vi "UI Main.vi"() -> ()   [LabVIEW 2012]
uses:
  controls/Control Configuration.ctl
  controls/UI Data.ctl
  controls/All FPGA Configuration Values.ctl
  controls/FPGA State.ctl
  controls/Raw Values.ctl
  Globals/Global - All UI Loop Stop.vi
  Globals/Global - UI Stream and Variable Connections.vi
  Globals/Global - Configuration Options.vi
  support/User Event - Stop/User Event - Stop.lvlib
  support/Message Queue/Message Queue.lvlib
panel:
  in  "Switch to Safe State":bool
  in  "Exit":bool
  out "System Status":string
  out "Current FPGA Control Mode":u16(ring) items=["Safe State", "Manual", "Control (PID)"]
  in  "Settings Tab":T1(tab)
  in  "Channel 3 Setpoint":fxp<+/-,16,5>
  in  "Channel 2 Setpoint":fxp<+/-,16,5>
  in  "Channel 1 Setpoint":fxp<+/-,16,5>
  in  "Channel 0 Setpoint":fxp<+/-,16,5>
  in  "Update Control Configuration":bool
  in  "Control Configurations":T2[](array[typedef])
  in  "Run Control":bool
  in  "Stop Control":bool
  in  "Channel 3 Manual Value":fxp<+/-,16,5>
  in  "Channel 2 Manual Value":fxp<+/-,16,5>
  in  "Channel 1 Manual Value":fxp<+/-,16,5>
  in  "Channel 0 Manual Value":fxp<+/-,16,5>
  in  "Run Manual":bool
  in  "Stop Manual":bool
  out "Input Values":T3(graph)
  out "Output Values":T3(graph)
  out "Actual Loop Period (ticks)":u32
  out "Largest Contiguous Memory (bytes)":dbl(graph)
  out "CPU Usage (%)":dbl(graph)
  out "Connected?":bool
  in  "Connect to Controller":bool
  in  "Controller Address":string
  # "LabVIEW FPGA Control on CompactRIO"
  # "Connection Settings"
  # "Element 0 - Chan 0\nElement 1 - Chan 1\nElement 2 - Chan 2\nElement 3 - Chan 3"
  # "Setpoint changes are sent to the target automatically."
  # "Control Configuration changes are sent to the target when you click \"Update Control Configurations\"."
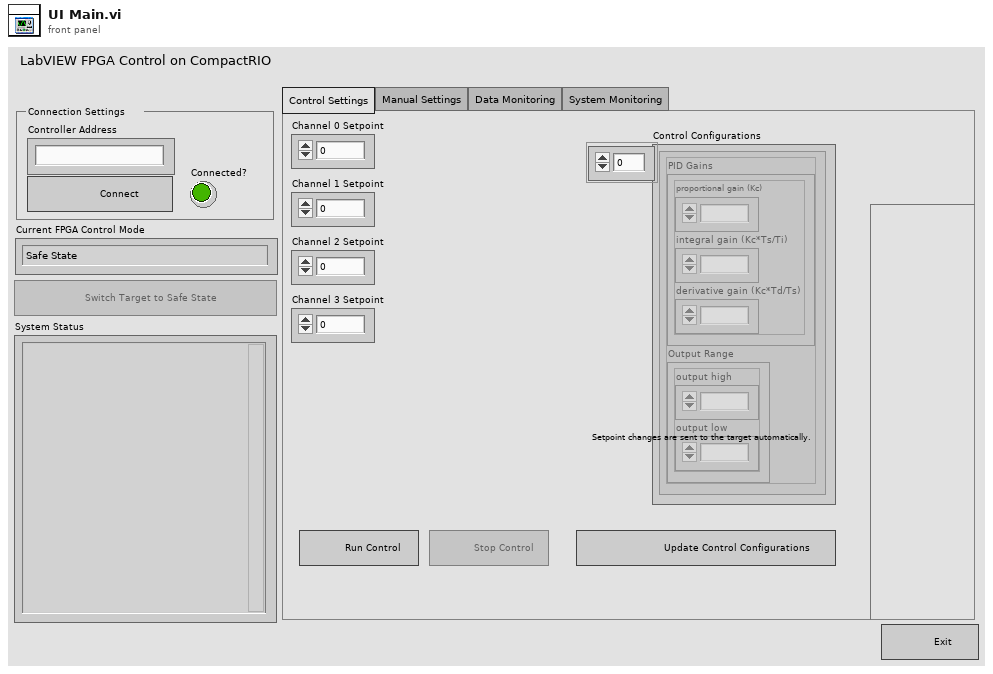
[diagram p1: front panel]
types:
  T1 = enum32{"Control Settings", "Manual Settings", "Data Monitoring", "System Monitoring"}
  T2 = typedef "Control Configuration.ctl" = cluster{"PID Gains":cluster{"proportional gain (Kc)":fxp<+/-,16,8>, "integral gain (Kc*Ts/Ti)":fxp<+/-,16,8>, "derivative gain (Kc*Td/Ts)":fxp<+/-,16,8>}, "Output Range":cluster{"output high":fxp<+/-,16,5>, "output low":fxp<+/-,16,5>}}
  T3 = cluster{"Channel 0":dbl, "Channel 1":dbl, "Channel 2":dbl, "Channel 3":dbl}
  T4 = typedef "UI Data.ctl" = cluster{"Switch to Safe State Ref":refnum<vi>, "Run Manual Ref":refnum<vi>, "Stop Manual Ref":refnum<vi>, "Run Control Ref":refnum<vi>, "Stop Control Ref":refnum<vi>, "Update Control Configurations Ref":refnum<vi>, "Ch 0 Setpoint Ref":refnum<vi>, "Ch 1 Setpoint Ref":refnum<vi>, "Ch 2 Setpoint Ref":refnum<vi>, "Ch 3 Setpoint Ref":refnum<vi>, "Ch 0 Manual Ref":refnum<vi>, "Ch 1 Manual Ref":refnum<vi>, "Ch 2 Manual Ref":refnum<vi>, "Ch 3 Manual Ref":refnum<vi>, "Control Configurations Ref":refnum<vi>}
  T5 = typedef "Message Queue.lvlib/All Message Queues.ctl" = cluster{"UI":refnum<queue>}
  T6 = cluster{"Channel 0 Setpoint":fxp<+/-,16,5>, "Channel 1 Setpoint":fxp<+/-,16,5>, "Channel 2 Setpoint":fxp<+/-,16,5>, "Channel 3 Setpoint":fxp<+/-,16,5>}
  T7 = cluster{"Channel 0 Manual Value":fxp<+/-,16,5>, "Channel 1 Manual Value":fxp<+/-,16,5>, "Channel 2 Manual Value":fxp<+/-,16,5>, "Channel 3 Manual Value":fxp<+/-,16,5>}
  T8 = cluster{"Message":string, "Message Data":variant}
  T9 = typedef "All FPGA Configuration Values.ctl" = cluster{"FPGA State":T10, "Manual Values":T11, "Setpoints":T11, "Control Configurations":T2[]}
  T10 = typedef "FPGA State.ctl" = enum16{"Safe State", "Manual", "Control (PID)"}
  T11 = typedef "Raw Values.ctl" = cluster{"Channel 0":fxp<+/-,20,5>, "Channel 1":fxp<+/-,20,5>, "Channel 2":fxp<+/-,20,5>, "Channel 3":fxp<+/-,20,5>}
  T12 = typedef "Variable References.ctl" = cluster{"CPU Usage":refnum<k21>, "Contiguous Memory":refnum<k21>, "Input Values":refnum<k21>, "Output Values":refnum<k21>, "FPGA Mode":refnum<k21>, "Actual Loop Period":refnum<k21>}
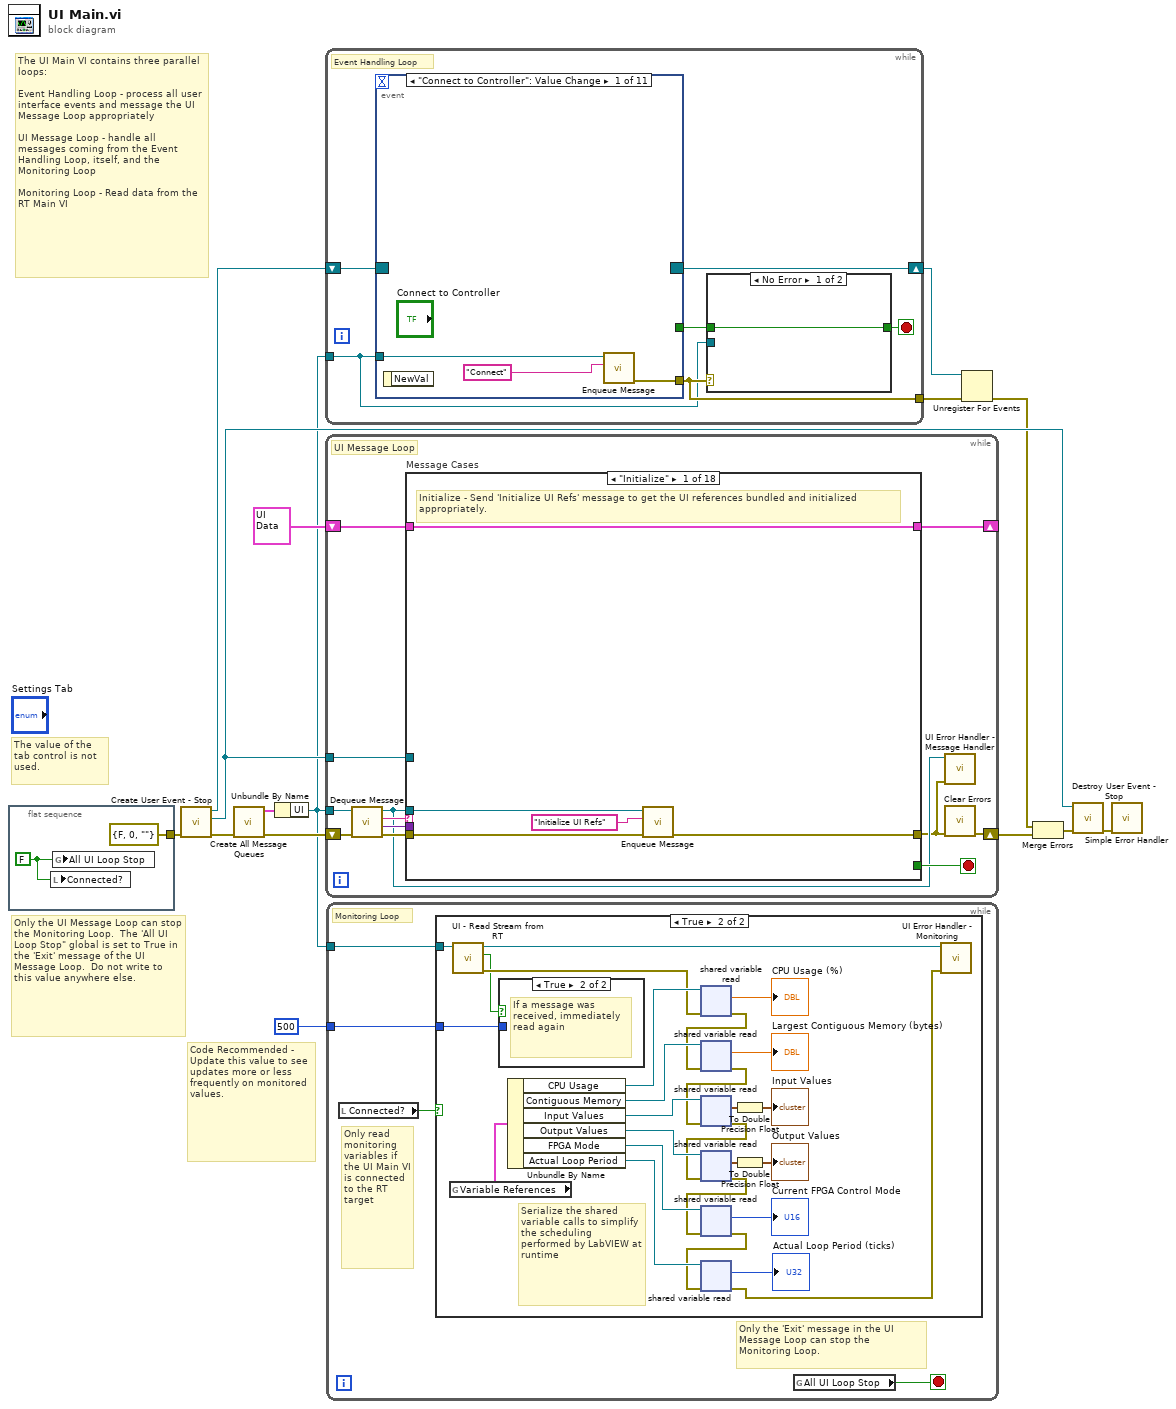
[diagram p0: block diagram]
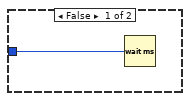
[diagram p2: hidden frame]
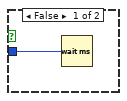
[diagram p3: hidden frame]
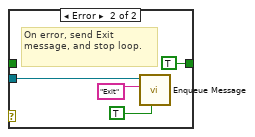
[diagram p4: hidden frame]
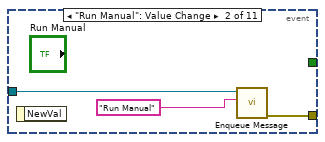
[diagram p5: hidden frame]
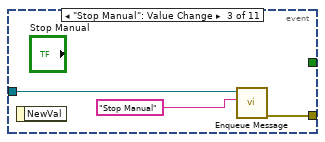
[diagram p6: hidden frame]
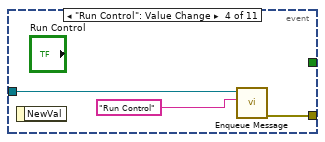
[diagram p7: hidden frame]
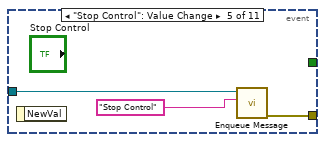
[diagram p8: hidden frame]
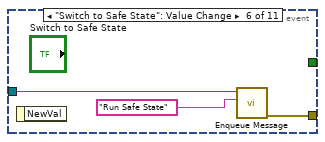
[diagram p9: hidden frame]
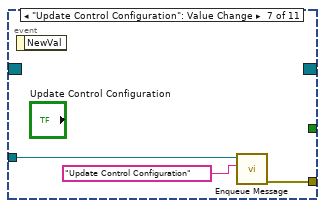
[diagram p10: hidden frame]
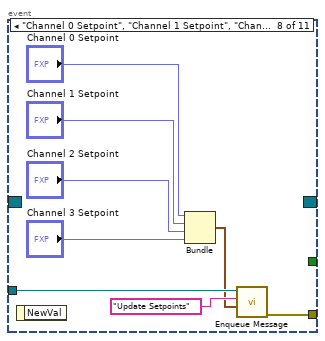
[diagram p11: hidden frame]
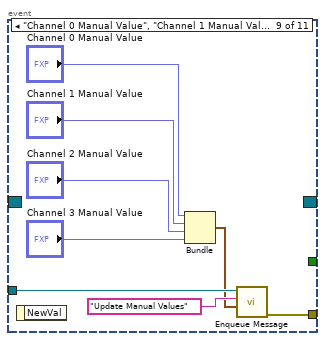
[diagram p12: hidden frame]
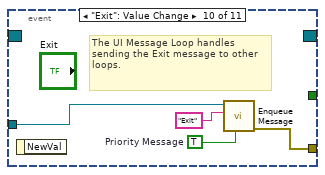
[diagram p13: hidden frame]
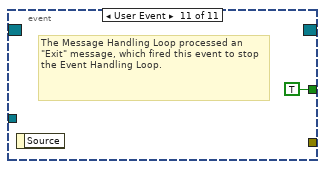
[diagram p14: hidden frame]
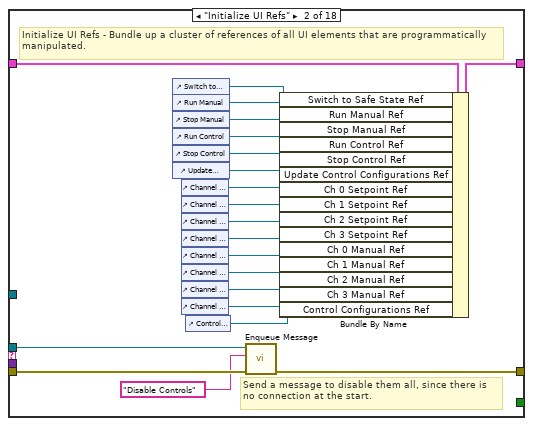
[diagram p15: hidden frame]
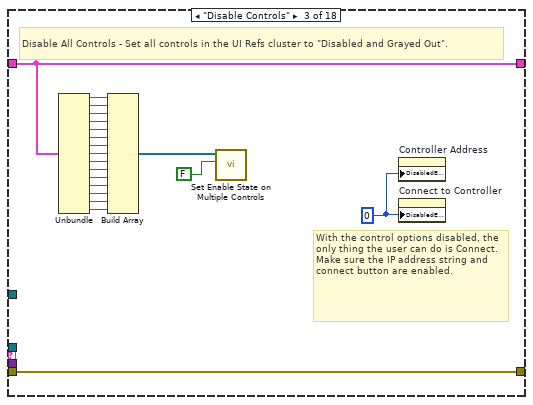
[diagram p16: hidden frame]
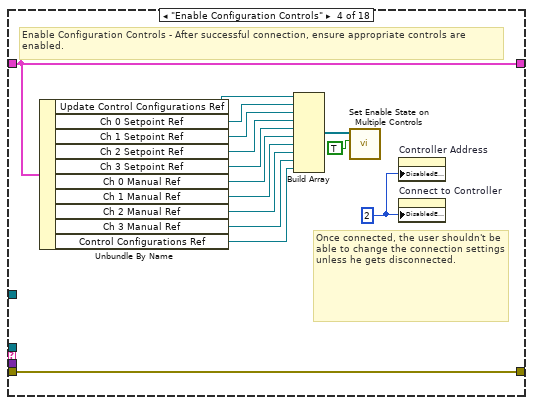
[diagram p17: hidden frame]
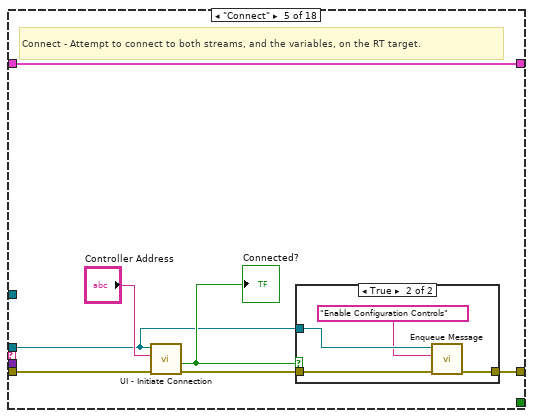
[diagram p18: hidden frame]
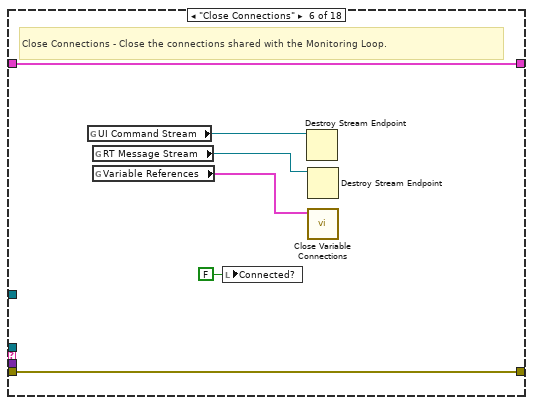
[diagram p20: hidden frame]
diagram:
  # "Code Recommended - Update this value to see updates more or less frequently on monitored values."
  # "The UI Main VI contains three parallel loops:\n\nEvent Handling Loop - process all user interface events and message the UI Message Loop appropriately\n\nUI Message Loop - handle all messages coming from the Event Handling Loop, itself, and the Monitoring Loop\n\nMonitoring Loop - Read data from the RT Main VI"
  # "The value of the tab control is not used."
  # "Only the UI Message Loop can stop the Monitoring Loop.  The 'All UI Loop Stop\" global is set to True in the 'Exit' message of the UI Message Loop.  Do not write to this value anywhere else."
  n1 = flat-sequence {
    tunnel: [errorcluster {"status"=FALSE, "code"=0, "source"=""} ("error in (no error)")] -> w2
    frame #0 {
      w16 = FALSE
      n2 = local write "Connected?"(w16) -> ()
      n3 = global write "Global - All UI Loop Stop.vi" "All UI Loop Stop"(w16) -> ()
    }
  }
  n4 = call "Create User Event - Stop.vi"("error in (no error)"=w2) -> ("error out"=w10:errorcluster, "User Event - Stop"=w11:refnum<user-event>, "Stop Event Registration Refnum"=w12:refnum<event-registration>)  [unwired: 8 in]
  n5 = call "Create All Message Queues.vi"("error in (no error)"=w10) -> ("error out"=w8:errorcluster, "Message Queues out"=w9:T5)  [unwired: 9 in]
  n6 = Unbundle By Name(w9) -> ("UI"=w3:refnum<queue>)
  n7 = while {
    tunnel: w3 -> [w19]
    tunnel: [w21] -> w14
    shift-right: [w18] -> w6
    shift-left: w12 -> [w20]
    stop <- w22 stop-if-true
    # "Event Handling Loop"
    n8 = event shown="[0] \"Connect to Controller\": Value Change" {
      selector: w20 -> [_ _ _ _ _ _ _ _ _ _ _]
      dyn-events: [_ _ _ _ _ _ _ _ _ _ _] -> w18
      timeout: _ -> [_ _ _ _ _ _ _ _ _ _ _]
      tunnel: [_ _ _ _ _ _ _ _ _ _ TRUE ("Discard?")] -> w23
      tunnel: w19 -> [w29 w32 w35 w38 w41 w44 w49 w52 w61 w66 _]
      tunnel: [w31 w34 w37 w40 w43 w46 w48 w51 w60 w69 _] -> w21
      event "Connect to Controller": Value Change {
        n9 = event-data() -> ()  [unwired: 1 in, 1 out]
        n10 = call "Enqueue Message.vi"("Message"="Connect", "Message Queue"=w29) -> ("error out"=w31:errorcluster)  [unwired: 8 in, 1 out]
      }
      event "Run Manual": Value Change {
        n11 = event-data() -> ()  [unwired: 1 in, 1 out]
        n12 = call "Enqueue Message.vi"("Message"="Run Manual", "Message Queue"=w32) -> ("error out"=w34:errorcluster)  [unwired: 8 in, 1 out]
      }
      event "Stop Manual": Value Change {
        n13 = event-data() -> ()  [unwired: 1 in, 1 out]
        n14 = call "Enqueue Message.vi"("Message"="Stop Manual", "Message Queue"=w35) -> ("error out"=w37:errorcluster)  [unwired: 8 in, 1 out]
      }
      event "Run Control": Value Change {
        n15 = event-data() -> ()  [unwired: 1 in, 1 out]
        n16 = call "Enqueue Message.vi"("Message"="Run Control", "Message Queue"=w38) -> ("error out"=w40:errorcluster)  [unwired: 8 in, 1 out]
      }
      event "Stop Control": Value Change {
        n17 = event-data() -> ()  [unwired: 1 in, 1 out]
        n18 = call "Enqueue Message.vi"("Message"="Stop Control", "Message Queue"=w41) -> ("error out"=w43:errorcluster)  [unwired: 8 in, 1 out]
      }
      event "Switch to Safe State": Value Change {
        n19 = event-data() -> ()  [unwired: 1 in, 1 out]
        n20 = call "Enqueue Message.vi"("Message"="Run Safe State", "Message Queue"=w44) -> ("error out"=w46:errorcluster)  [unwired: 8 in, 1 out]
      }
      event "Update Control Configuration": Value Change {
        n21 = event-data() -> ()  [unwired: 1 in, 1 out]
        n22 = call "Enqueue Message.vi"("Message"="Update Control Configuration", "Message Queue"=w49) -> ("error out"=w48:errorcluster)  [unwired: 8 in, 1 out]
      }
      event "Channel 0 Setpoint", "Channel 1 Setpoint", "Channel 2 Setpoint", "Channel 3 Setpoint": Value Change {
        n23 = event-data() -> ()  [unwired: 1 in, 1 out]
        n24 = Bundle("Channel 0 Setpoint"="Channel 0 Setpoint", "Channel 1 Setpoint"="Channel 1 Setpoint", "Channel 2 Setpoint"="Channel 2 Setpoint", "Channel 3 Setpoint"="Channel 3 Setpoint") -> (w50:T6)  [unwired: 1 in]
        n25 = call "Enqueue Message.vi"("Message Data"=w50, "Message"="Update Setpoints", "Message Queue"=w52) -> ("error out"=w51:errorcluster)  [unwired: 7 in, 1 out]
      }
      event "Channel 0 Manual Value", "Channel 1 Manual Value", "Channel 2 Manual Value", "Channel 3 Manual Value": Value Change {
        n26 = event-data() -> ()  [unwired: 1 in, 1 out]
        n27 = Bundle("Channel 0 Manual Value"="Channel 0 Manual Value", "Channel 1 Manual Value"="Channel 1 Manual Value", "Channel 2 Manual Value"="Channel 2 Manual Value", "Channel 3 Manual Value"="Channel 3 Manual Value") -> (w58:T7)  [unwired: 1 in]
        n28 = call "Enqueue Message.vi"("Message Data"=w58, "Message"="Update Manual Values", "Message Queue"=w61) -> ("error out"=w60:errorcluster)  [unwired: 7 in, 1 out]
      }
      event "Exit": Value Change {
        w67 = TRUE  # Priority Message
        # "The UI Message Loop handles sending the Exit message to other loops."
        n29 = event-data() -> ()  [unwired: 1 in, 1 out]
        n30 = call "Enqueue Message.vi"("Priority Message? (F)"=w67, "Message"="Exit", "Message Queue"=w66) -> ("error out"=w69:errorcluster)  [unwired: 7 in, 1 out]
      }
      event User Event {
        # "The Message Handling Loop processed an \"Exit\" message, which fired this event to stop the Event Handling Loop."
        n31 = event-data() -> ()  [unwired: 1 in, 1 out]
      }
    }
    n32 = case shown="No Error" w21 {
      tunnel: [w24 TRUE ("Discard?")] -> w22
      tunnel: w23 -> [w24 _]
      tunnel: w19 -> [_ w25]
      frame No Error {
      }
      frame Error {
        # "On error, send Exit message, and stop loop."
        n33 = call "Enqueue Message.vi"("Priority Message? (F)"=TRUE ("Discard?"), "Message"="Exit", "Message Queue"=w25) -> ()  [unwired: 7 in, 2 out]
      }
    }
  }
  n34 = while {
    tunnel: w3 -> [w76]
    tunnel: w11 -> [w81]
    shift-right: [w71] -> w15
    shift-left: w8 -> [w80]
    shift-right: [w74] -> _
    shift-left: T4 {"Switch to Safe State Ref"=refnum, "Run Manual Ref"=refnum, "Stop Manual Ref"=refnum, "Run Control Ref"=refnum, "Stop Control Ref"=refnum, "Update Control Configurations Ref"=refnum, "Ch 0 Setpoint Ref"=refnum, "Ch 1 Setpoint Ref"=refnum, "Ch 2 Setpoint Ref"=refnum, "Ch 3 Setpoint Ref"=refnum, "Ch 0 Manual Ref"=refnum, "Ch 1 Manual Ref"=refnum, "Ch 2 Manual Ref"=refnum, "Ch 3 Manual Ref"=refnum, "Control Configurations Ref"=refnum} ("Measurement UI Controls") -> [w75]
    stop <- w82 stop-if-true
    # "UI Message Loop"
    n35 = call "Dequeue Message.vi"("error in (no error)"=w80, "Message Queue"=w76) -> ("error out"=w79:errorcluster, "Message Data"=w77:variant, "Message"=w78:string, "dup Message Queue"=w73:refnum<queue>)  [unwired: 6 in]
    n36 = case "Message Cases" shown="\"Initialize\"" w78 {
      selector: w78 -> [_ _ _ _ _ _ _ _ _ w205 _ w237 _ w287 _ _ _ w348]
      tunnel: w73 -> [w84 w89 _ _ w145 _ w163 _ w177 w206 _ _ _ w291 _ w333 _ _]
      tunnel: w79 -> [w86 w108 w128 w129 w150 w161 w165 w170 w201 w208 w226 w238 w258 w301 w322 w338 w343 _]
      tunnel: [w85 w90 w128 w129 w144 w161 w164 w169 w180 w207 w225 w239 w257 w302 w320 w339 w342 w346] -> w72
      tunnel: [_ _ _ _ _ _ _ _ _ _ _ _ _ _ _ TRUE _ _] -> w82
      tunnel: w77 -> [_ _ _ _ _ _ _ _ w199 _ _ w236 w256 w299 w319 _ _ _]
      tunnel: w81 -> [_ _ _ _ _ _ _ _ _ _ _ _ _ _ _ w337 _ _]
      tunnel: w75 -> [w87 w107 w127 w140 w149 w160 w167 w171 w196 w209 w227 w240 w255 w303 w321 w335 w341 w344]
      tunnel: [w87 w106 w127 w140 w149 w160 w167 w171 w196 w209 w227 w240 w255 w303 w321 w335 w341 w344] -> w74
      frame "Initialize" {
        # "Initialize - Send 'Initialize UI Refs' message to get the UI references bundled and initialized appropriately."
        n37 = call "Enqueue Message.vi"("error in (no error)"=w86, "Message"="Initialize UI Refs", "Message Queue"=w84) -> ("error out"=w85:errorcluster)  [unwired: 7 in, 1 out]
      }
      frame "Initialize UI Refs" {
        # "Send a message to disable them all, since there is no connection at the start."
        # "Initialize UI Refs - Bundle up a cluster of references of all UI elements that are programmatically manipulated."
        n38 = control-ref of="Switch to Safe State"() -> (w105:refnum<vi>)
        n39 = control-ref of="Run Manual"() -> (w104:refnum<vi>)
        n40 = control-ref of="Stop Manual"() -> (w103:refnum<vi>)
        n41 = control-ref of="Run Control"() -> (w102:refnum<vi>)
        n42 = control-ref of="Stop Control"() -> (w101:refnum<vi>)
        n43 = control-ref of="Update Control Configuration"() -> (w100:refnum<vi>)
        n44 = control-ref of="Channel 0 Setpoint"() -> (w99:refnum<vi>)
        n45 = control-ref of="Channel 1 Setpoint"() -> (w98:refnum<vi>)
        n46 = control-ref of="Channel 2 Setpoint"() -> (w97:refnum<vi>)
        n47 = control-ref of="Channel 3 Setpoint"() -> (w96:refnum<vi>)
        n48 = control-ref of="Channel 0 Manual Value"() -> (w95:refnum<vi>)
        n49 = control-ref of="Channel 1 Manual Value"() -> (w94:refnum<vi>)
        n50 = control-ref of="Channel 2 Manual Value"() -> (w93:refnum<vi>)
        n51 = control-ref of="Channel 3 Manual Value"() -> (w92:refnum<vi>)
        n52 = control-ref of="Control Configurations"() -> (w91:refnum<vi>)
        n53 = call "Enqueue Message.vi"("error in (no error)"=w108, "Message"="Disable Controls", "Message Queue"=w89) -> ("error out"=w90:errorcluster)  [unwired: 7 in, 1 out]
        n54 = Bundle By Name(cluster=w107, "Switch to Safe State Ref"=w105, "Run Manual Ref"=w104, "Stop Manual Ref"=w103, "Run Control Ref"=w102, "Stop Control Ref"=w101, "Update Control Configurations Ref"=w100, "Ch 0 Setpoint Ref"=w99, "Ch 1 Setpoint Ref"=w98, "Ch 2 Setpoint Ref"=w97, "Ch 3 Setpoint Ref"=w96, "Ch 0 Manual Ref"=w95, "Ch 1 Manual Ref"=w94, "Ch 2 Manual Ref"=w93, "Ch 3 Manual Ref"=w92, "Control Configurations Ref"=w91) -> (w106:T4)
      }
      frame "Disable Controls" {
        w109 = 0
        # "With the control options disabled, the only thing the user can do is Connect. Make sure the IP address string and connect button are enabled."
        # "Disable All Controls - Set all controls in the UI Refs cluster to \"Disabled and Grayed Out\"."
        n55 = Unbundle(w127) -> ("Switch to Safe State Ref"=w126:refnum<vi>, "Run Manual Ref"=w125:refnum<vi>, "Stop Manual Ref"=w124:refnum<vi>, "Run Control Ref"=w123:refnum<vi>, "Stop Control Ref"=w122:refnum<vi>, "Update Control Configurations Ref"=w121:refnum<vi>, "Ch 0 Setpoint Ref"=w120:refnum<vi>, "Ch 1 Setpoint Ref"=w119:refnum<vi>, "Ch 2 Setpoint Ref"=w118:refnum<vi>, "Ch 3 Setpoint Ref"=w117:refnum<vi>, "Ch 0 Manual Ref"=w116:refnum<vi>, "Ch 1 Manual Ref"=w115:refnum<vi>, "Ch 2 Manual Ref"=w114:refnum<vi>, "Ch 3 Manual Ref"=w113:refnum<vi>, "Control Configurations Ref"=w112:refnum<vi>)
        n56 = Build Array(w126, w125, w124, w123, w122, w121, w120, w119, w118, w117, w116, w115, w114, w113, w112) -> (w111:refnum<vi>[])
        n57 = call "Set Enable State on Multiple Controls.vi"("Enable?"=FALSE, "Controls"=w111) -> ()  [unwired: 10 in]
        n58 = property on="Controller Address" class="Str"("DisabledEnum"=w109) -> ()  [unwired: 2 in, 2 out]
        n59 = property on="Connect to Controller" class="Bool"("DisabledEnum"=w109) -> ()  [unwired: 2 in, 2 out]
      }
      frame "Enable Configuration Controls" {
        w141 = 2
        # "Once connected, the user shouldn't be able to change the connection settings unless he gets disconnected."
        # "Enable Configuration Controls - After successful connection, ensure appropriate controls are enabled."
        n60 = Unbundle By Name(w140) -> ("Update Control Configurations Ref"=w139:refnum<vi>, "Ch 0 Setpoint Ref"=w138:refnum<vi>, "Ch 1 Setpoint Ref"=w137:refnum<vi>, "Ch 2 Setpoint Ref"=w136:refnum<vi>, "Ch 3 Setpoint Ref"=w135:refnum<vi>, "Ch 0 Manual Ref"=w134:refnum<vi>, "Ch 1 Manual Ref"=w133:refnum<vi>, "Ch 2 Manual Ref"=w132:refnum<vi>, "Ch 3 Manual Ref"=w131:refnum<vi>, "Control Configurations Ref"=w130:refnum<vi>)
        n61 = Build Array(w139, w138, w137, w136, w135, w134, w133, w132, w131, w130) -> (w143:refnum<vi>[])
        n62 = call "Set Enable State on Multiple Controls.vi"("Enable?"=TRUE, "Controls"=w143) -> ()  [unwired: 10 in]
        n63 = property on="Controller Address" class="Str"("DisabledEnum"=w141) -> ()  [unwired: 2 in, 2 out]
        n64 = property on="Connect to Controller" class="Bool"("DisabledEnum"=w141) -> ()  [unwired: 2 in, 2 out]
      }
      frame "Connect" {
        # "Connect - Attempt to connect to both streams, and the variables, on the RT target."
        n65 = call "UI - Initiate Connection.vi"("error in (no error)"=w150, "Controller Address"="Controller Address", "Message Queue"=w145) -> ("error out"=w147:errorcluster, "Connected?"=w146:bool)  [unwired: 7 in]
        "Connected?" <- w146
        n66 = case shown="True" w146 {
          tunnel: w147 -> [w151 w155]
          tunnel: w145 -> [_ w154]
          tunnel: [w151 w153] -> w144
          frame False {
          }
          frame True {
            n67 = call "Enqueue Message.vi"("error in (no error)"=w155, "Message"="Enable Configuration Controls", "Message Queue"=w154) -> ("error out"=w153:errorcluster)  [unwired: 7 in, 1 out]
          }
        }
      }
      frame "Close Connections" {
        # "Close Connections - Close the connections shared with the Monitoring Loop."
        n68 = global read "Global - UI Stream and Variable Connections.vi" "UI Command Stream"() -> (w159:refnum<k21>)
        n69 = global read "Global - UI Stream and Variable Connections.vi" "RT Message Stream"() -> (w158:refnum<k21>)
        n70 = global read "Global - UI Stream and Variable Connections.vi" "Variable References"() -> (w157:T12)
        n71 = local write "Connected?"(FALSE ("Connected?")) -> ()
        n72 = Destroy Stream Endpoint(11:w159) -> ()  [unwired: 1 in, 1 out]
        n73 = Destroy Stream Endpoint(11:w158) -> ()  [unwired: 1 in, 1 out]
        n74 = call "Close Variable Connections.vi"("Variable References"=w157) -> ()  [unwired: 11 in]
      }
      frame "Disconnect UI" {
        # "Disconnect UI - Something has gone wrong with the connection. Reinitialize the UI to its disconnected state."
        n75 = local write "Connected?"(FALSE ("Connected?")) -> ()
        n76 = call "Enqueue Message.vi"("error in (no error)"=w165, "Message"="Disable Controls", "Message Queue"=w163) -> ("error out"=w164:errorcluster)  [unwired: 7 in, 1 out]
      }
      frame "Get Settings from FPGA" {
        # "Get Settings from FPGA - Send a command to the RT to retrieve all current FPGA Main VI parameter values and send them back to the UI."
        n77 = local read "Connected?"() -> (w168:bool)
        n78 = case shown="True" w168 {
          tunnel: w170 -> [w172 w176]
          tunnel: [w172 w175] -> w169
          frame False {
            # "Don't bother trying to send a message to the RT system if UI Main VI isn't even connected"
          }
          frame True {
            n79 = global read "Global - UI Stream and Variable Connections.vi" "UI Command Stream"() -> (w173:refnum<k21>)
            n80 = shared-variable-write(w173, w176, T8 {"Message"="Send FPGA Configuration to UI", "Message Data"=variant} ("data in")) -> (w175:errorcluster)  [unwired: 1 in, 2 out]
          }
        }
      }
      frame "Initial UI Values" {
        # "Initial UI Values - These are the current values of the FPGA Main VI's R/W controls. They are used to initialize the panel of UI Main VI upon successful connection to the RT target."
        # "Set values of all manual and setpoint controls via reference."
        n81 = Variant To Data(error in=w201, type=T9 {"FPGA State"=enum."Safe State", "Manual Values"={"Channel 0"=0.0, "Channel 1"=0.0, "Channel 2"=0.0, "Channel 3"=0.0}, "Setpoints"={"Channel 0"=0.0, "Channel 1"=0.0, "Channel 2"=0.0, "Channel 3"=0.0}, "Control Configurations"=[]} ("All FPGA Configuration Values"), Variant=w199) -> (data=w197:T9, error out=w200:errorcluster)
        n82 = Unbundle By Name(w196) -> ("Ch 0 Setpoint Ref"=w191:refnum<vi>, "Ch 1 Setpoint Ref"=w190:refnum<vi>, "Ch 2 Setpoint Ref"=w189:refnum<vi>, "Ch 3 Setpoint Ref"=w188:refnum<vi>, "Ch 0 Manual Ref"=w187:refnum<vi>, "Ch 1 Manual Ref"=w186:refnum<vi>, "Ch 2 Manual Ref"=w185:refnum<vi>, "Ch 3 Manual Ref"=w184:refnum<vi>)
        n83 = Unbundle By Name(w197) -> ("Setpoints"=w195:T11, "Manual Values"=w194:T11, "Control Configurations"=w181:T2[], "FPGA State"=w178:T10)
        n84 = Build Array(w191, w190, w189, w188, w187, w186, w185, w184) -> (w183:refnum<vi>[])
        n85 = Cluster To Array(cluster=w195) -> (array=w193:fxp<+/-,20,5>[])
        n86 = Cluster To Array(cluster=w194) -> (array=w192:fxp<+/-,20,5>[])
        n87 = local write "Current FPGA Control Mode"(w178) -> ()
        n88 = Build Array (concatenate)(w193, w192) -> (w182:fxp<+/-,20,5>[])
        n89 = local write "Control Configurations"(w181) -> ()
        n90 = for {
          tunnel: w183 -> [w203] mode=indexing
          tunnel: w182 -> [w202] mode=indexing
          n91 = property class="DigNum"(reference=w203, "Value"=w202) -> ()  [unwired: 1 in, 2 out]
        }
        n92 = call "Enqueue Message.vi"("error in (no error)"=w200, "Message Data"=w178, "Message"="Update Display Mode", "Message Queue"=w177) -> ("error out"=w180:errorcluster)  [unwired: 6 in, 1 out]
      }
      frame "Run Control", "Run Manual", "Run Safe State", "Stop Control", "Stop Manual" {
        # "Run/Stop buttons - Send a command to switch the FPGA into the appropriate state. Send a message to update this UI to reflect the new state."
        n93 = local read "Connected?"() -> (w204:bool)
        n94 = case shown="True" w204 {
          tunnel: w208 -> [w210 w220]
          tunnel: [w210 w216] -> w207
          tunnel: w206 -> [_ w215]
          tunnel: w205 -> [_ w214]
          frame False {
            # "Don't bother trying to send a message to the RT system if UI Main VI isn't even connected"
          }
          frame True {
            # "Run Manual and Run Control switch into their respective states. Anything else switches to Safe State."
            n95 = case shown="\"Safe State\", \"Stop Control\", \"Stop Manual\", Default" w214 {
              tunnel: [FPGA_State."Safe State" ("FPGA State") FPGA_State."Control (PID)" ("FPGA State") FPGA_State."Manual" ("FPGA State")] -> w211
              frame "Safe State", "Stop Control", "Stop Manual", Default {
              }
              frame "Run Control" {
              }
              frame "Run Manual" {
              }
            }
            n96 = global read "Global - UI Stream and Variable Connections.vi" "UI Command Stream"() -> (w212:refnum<k21>)
            n97 = Bundle("Update FPGA State", "FPGA State"=w211) -> (w217:cluster{string, "FPGA State":T10})  [unwired: 1 in]
            n98 = shared-variable-write(w212, w220, w217) -> (w219:errorcluster)  [unwired: 1 in, 2 out]
            n99 = call "Enqueue Message.vi"("error in (no error)"=w219, "Message Data"=w211, "Message"="Update Display Mode", "Message Queue"=w215) -> ("error out"=w216:errorcluster)  [unwired: 6 in, 1 out]
          }
        }
      }
      frame "Update Control Configuration" {
        # "Update Control Configuration - Send all control configurations to RT to be sent down to the FPGA."
        n100 = local read "Connected?"() -> (w224:bool)
        n101 = case shown="True" w224 {
          tunnel: w226 -> [w228 w234]
          tunnel: [w228 w233] -> w225
          frame False {
            # "Don't bother trying to send a message to the RT system if UI Main VI isn't even connected"
          }
          frame True {
            n102 = global read "Global - UI Stream and Variable Connections.vi" "UI Command Stream"() -> (w229:refnum<k21>)
            n103 = Bundle("Update Control Configurations", "Control Configurations"="Control Configurations") -> (w231:cluster{string, "Control Configurations":T2[]})  [unwired: 1 in]
            n104 = shared-variable-write(w229, w234, w231) -> (w233:errorcluster)  [unwired: 1 in, 2 out]
          }
        }
      }
      frame "Update Manual Values", "Update Setpoints" {
        # "Update Manual Values/Setpoints - Send all manual values/setpoints to RT to be sent down to the FPGA."
        n105 = local read "Connected?"() -> (w235:bool)
        n106 = case shown="True" w235 {
          tunnel: [w241 w247] -> w239
          tunnel: w238 -> [w241 w245]
          tunnel: w237 -> [_ w244]
          tunnel: w236 -> [_ w243]
          frame False {
            # "Don't bother trying to send a message to the RT system if UI Main VI isn't even connected"
          }
          frame True {
            n107 = global read "Global - UI Stream and Variable Connections.vi" "UI Command Stream"() -> (w242:refnum<k21>)
            n108 = Bundle(w244, "Message Data"=w243) -> (w246:cluster{string, "Message Data":variant})  [unwired: 1 in]
            n109 = shared-variable-write(w242, w245, w246) -> (w247:errorcluster)  [unwired: 1 in, 2 out]
          }
        }
      }
      frame "Update Display Mode" {
        # "Update Display Mode - Enable/Disable Controls appropriately for the new display mode."
        n110 = Variant To Data(error in=w258, type=FPGA_State."Safe State" ("FPGA State"), Variant=w256) -> (data=w254:T10, error out=w257:errorcluster)
        n111 = Unbundle By Name(w255) -> ("Switch to Safe State Ref"=w253:refnum<vi>, "Run Manual Ref"=w252:refnum<vi>, "Stop Manual Ref"=w251:refnum<vi>, "Run Control Ref"=w250:refnum<vi>, "Stop Control Ref"=w249:refnum<vi>)
        n112 = case shown="\"Manual\"" w254 {
          tunnel: w253 -> [w263 w272 w279]
          tunnel: w252 -> [w259 w271 w281]
          tunnel: w251 -> [w262 w270 w278]
          tunnel: w250 -> [w261 w268 w280]
          tunnel: w249 -> [w260 w269 w277]
          frame "Control (PID)" {
            n113 = Build Array "Controls to Enable"(w263, w260, w259) -> (w267:refnum<vi>[])
            n114 = Build Array "Controls to Disable"(w262, w261) -> (w265:refnum<vi>[])
            n115 = call "Set Enable State on Multiple Controls.vi"("Enable?"=FALSE, "Controls"=w265) -> ()  [unwired: 10 in]
            n116 = call "Set Enable State on Multiple Controls.vi"("Enable?"=TRUE, "Controls"=w267) -> ()  [unwired: 10 in]
          }
          frame "Manual" {
            n117 = Build Array "Controls to Enable"(w272, w270, w268) -> (w276:refnum<vi>[])
            n118 = Build Array "Controls to Disable"(w271, w269) -> (w274:refnum<vi>[])
            n119 = call "Set Enable State on Multiple Controls.vi"("Enable?"=FALSE, "Controls"=w274) -> ()  [unwired: 10 in]
            n120 = call "Set Enable State on Multiple Controls.vi"("Enable?"=TRUE, "Controls"=w276) -> ()  [unwired: 10 in]
          }
          frame "Safe State" {
            # "This frame runs when FPGA is in Safe State. Only enable the two run buttons."
            n121 = Build Array "Controls to Enable"(w281, w280) -> (w285:refnum<vi>[])
            n122 = Build Array "Controls to Disable"(w279, w278, w277) -> (w283:refnum<vi>[])
            n123 = call "Set Enable State on Multiple Controls.vi"("Enable?"=FALSE, "Controls"=w283) -> ()  [unwired: 10 in]
            n124 = call "Set Enable State on Multiple Controls.vi"("Enable?"=TRUE, "Controls"=w285) -> ()  [unwired: 10 in]
          }
        }
      }
      frame "Critical Error", "Log-Only Error", "Non-Critical Error", "RT Error" {
        # "Error - Display message in status indicator on panel.  If it's a critical error, shut down this VI with an 'Exit' message."
        n125 = case shown="Default" w287 {
          selector: w287 -> [_ w305]
          tunnel: ["UI Error" w305] -> w286
          frame Default {
          }
          frame "RT Error" {
          }
        }
        n126 = Variant To Data(error in=w301, type=errorcluster {"status"=FALSE, "code"=0, "source"=""} ("error constant"), Variant=w299) -> (data=w294:errorcluster, error out=w300:errorcluster)
        n127 = Unbundle By Name(w294) -> ("code"=w293:i32, "source"=w297:string)
        n128 = Format Date/Time String() -> (date/time string=w296:string)  [unwired: 3 in]
        n129 = Format Into String(format string="\n%s: %s %d - %s", w296, w286, w293, w297) -> (resulting string=w288:string)  [unwired: 2 in, 1 out]
        n130 = call "Enqueue Message.vi"("error in (no error)"=w300, "Message Data"=w288, "Message"="Update System Status", "Message Queue"=w291) -> ("error out"=w292:errorcluster, "dup Message Queue"=w290:refnum<queue>)  [unwired: 6 in]
        n131 = case shown="Default" w287 {
          tunnel: w292 -> [w306 w310]
          tunnel: w290 -> [_ w308]
          tunnel: [w306 w309] -> w302
          frame Default {
          }
          frame "Critical Error" {
            n132 = call "Enqueue Message.vi"("error in (no error)"=w310, "Message"="Exit", "Message Queue"=w308) -> ("error out"=w309:errorcluster)  [unwired: 7 in, 1 out]
          }
        }
      }
      frame "Update System Status" {
        # "Code Recommended - The code below ensures that the System Status string value does not become too large.  It uses the same maximum size as the RT error log to determine whether or not to remove the last half of the log string. Change this logic if you wish to maintain more/less of the information in the System Status string."
        # "Update System Status - Add a new string to the beginning of the System Status string on the UI."
        n133 = Variant To Data(error in=w322, type="", Variant=w319) -> (data=w316:string, error out=w320:errorcluster)
        n134 = local read "System Status"() -> (w314:string)
        n135 = global read "Global - Configuration Options.vi" "Error Log Max Size (bytes)"() -> (w312:i64)
        n136 = String Length(string=w314) -> (length=w315:i32)
        n137 = Greater?(x=w315, y=w312) -> (0:w313:bool)
        n138 = case shown="True" w313 {
          tunnel: w314 -> [w323 w327]
          tunnel: w312 -> [_ w326]
          tunnel: [w323 w328] -> w311
          frame False {
          }
          frame True {
            n139 = Divide(x=w326, y=i64 2) -> (x/y=w325:dbl)
            n140 = String Subset(string=w327, length (rest)=w325) -> (substring=w328:string)  [unwired: 1 in]
          }
        }
        n141 = Concatenate Strings(w316, w311) -> (→"System Status":string)
      }
      frame "Exit" {
        # "Close all connections"
        # "Stop Monitoring Loop"
        # "Stop Event Handling Loop"
        # "Release the UI Message queue reference"
        # "Stop UI Message Loop"
        # "Exit - Fire the User Event to stop the Event Handling Loop, and toggle the local variable to stop the Monitoring Loop.  This message alone causes all three loops to stop."
        n142 = global write "Global - All UI Loop Stop.vi" "All UI Loop Stop"(TRUE ("Stop Monitoring Loop")) -> ()
        n143 = call "Fire User Event - Stop.vi"("User Event - Stop"=w337) -> ("error out"=w336:errorcluster)  [unwired: 10 in]
        n144 = Release Queue(queue=w333, error in (no error)=w338) -> (error out=w334:errorcluster)  [unwired: 1 in, 2 out]
        n145 = global read "Global - UI Stream and Variable Connections.vi" "UI Command Stream"() -> (w331:refnum<k21>)
        n146 = global read "Global - UI Stream and Variable Connections.vi" "RT Message Stream"() -> (w330:refnum<k21>)
        n147 = global read "Global - UI Stream and Variable Connections.vi" "Variable References"() -> (w329:T12)
        n148 = Destroy Stream Endpoint(11:w331) -> ()  [unwired: 1 in, 1 out]
        n149 = Destroy Stream Endpoint(11:w330) -> ()  [unwired: 1 in, 1 out]
        n150 = call "Close Variable Connections.vi"("Variable References"=w329) -> ()  [unwired: 11 in]
        n151 = Merge Errors(w336, w334) -> (w339:errorcluster)
      }
      frame "---Copy This Frame---" {
        # "Duplicate this frame when creating new messages.  Change this comment in the duplicated frame to describe this message."
        n152 = Merge Errors(w343) -> (w342:errorcluster)
      }
      frame Default {
        # "'Default' case only runs if there is a message that isn't defined in any of the other cases.  Output a programming error."
        n153 = Format Into String(format string="The invalid message string \"%s\" was received in the Message Handling Loop." ("Invalid Message Loop Message"), w348) -> (resulting string=w345:string)  [unwired: 2 in, 1 out]
        n154 = call <vilib>:"Error Cluster From Error Code.vi"("error message (\"\")"=w345, "error code (0)"=1) -> ("error out"=w346:errorcluster)  [unwired: 7 in]
      }
    }
    n155 = call "UI Error Handler - Message Handler.vi"("error in (no error)"=w72, "Message Queue"=w73) -> ()  [unwired: 9 in, 1 out]
    n156 = call <vilib>:"Clear Errors.vi"("error in (no error)"=w72) -> ("error out"=w71:errorcluster)  [unwired: 6 in]
  }
  n157 = while {
    tunnel: w3 -> [w352]
    tunnel: u32 500 ("milliseconds to wait") -> [w350]
    stop <- w353 stop-if-true
    # "Only read monitoring variables if the UI Main VI is connected to the RT target"
    # "Only the 'Exit' message in the UI Message Loop can stop the Monitoring Loop."
    # "Monitoring Loop"
    n158 = local read "Connected?"() -> (w351:bool)
    n159 = case shown="True" w351 {
      tunnel: w352 -> [_ w360]
      tunnel: w350 -> [w354 w355]
      frame False {
        n160 = Wait (ms)(milliseconds to wait=w354) -> ()  [unwired: 1 out]
      }
      frame True {
        # "Serialize the shared variable calls to simplify the scheduling performed by LabVIEW at runtime"
        n161 = global read "Global - UI Stream and Variable Connections.vi" "Variable References"() -> (w358:T12)
        n162 = call "UI - Read Stream from RT.vi"("Message Queue"=w360) -> ("error out"=w366:errorcluster, "Message Received?"=w356:bool, "dup Message Queue"=w359:refnum<queue>)  [unwired: 8 in]
        n163 = case shown="True" w356 {
          tunnel: w355 -> [w381 _]
          frame False {
            n164 = Wait (ms)(milliseconds to wait=w381) -> ()  [unwired: 1 out]
          }
          frame True {
            # "If a message was received, immediately read again"
          }
        }
        n165 = Unbundle By Name(w358) -> ("CPU Usage"=w373:refnum<k21>, "Contiguous Memory"=w372:refnum<k21>, "Input Values"=w371:refnum<k21>, "Output Values"=w370:refnum<k21>, "FPGA Mode"=w369:refnum<k21>, "Actual Loop Period"=w368:refnum<k21>)
        n166 = shared-variable-read(w373, w366) -> (w365:errorcluster, →"CPU Usage (%)":dbl)  [unwired: 2 out]
        n167 = shared-variable-read(w372, w365) -> (w364:errorcluster, →"Largest Contiguous Memory (bytes)":dbl)  [unwired: 2 out]
        n168 = shared-variable-read(w371, w364) -> (w363:errorcluster, w376:T11)  [unwired: 2 out]
        n169 = shared-variable-read(w370, w363) -> (w362:errorcluster, w375:T11)  [unwired: 2 out]
        n170 = shared-variable-read(w369, w362) -> (w361:errorcluster, →"Current FPGA Control Mode":T10)  [unwired: 2 out]
        n171 = shared-variable-read(w368, w361) -> (w367:errorcluster, →"Actual Loop Period (ticks)":u32)  [unwired: 2 out]
        n172 = To Double Precision Float(number=w376) -> (double precision float=→"Input Values":T3)
        n173 = To Double Precision Float(number=w375) -> (double precision float=→"Output Values":T3)
        n174 = call "UI Error Handler - Monitoring.vi"("error in (no error)"=w367, "Message Queue"=w359) -> ()  [unwired: 9 in, 1 out]
      }
    }
    n175 = global read "Global - All UI Loop Stop.vi" "All UI Loop Stop"() -> (w353:bool)
  }
  n176 = Unregister For Events(event registration refnum=w6, error in=w14) -> (error out=w7:errorcluster)
  n177 = Merge Errors(w7, w15) -> (w13:errorcluster)
  n178 = call "Destroy User Event - Stop.vi"("error in (no error)"=w13, "User Event - Stop"=w11) -> ("error out"=w4:errorcluster)  [unwired: 9 in]
  n179 = call <vilib>:"Simple Error Handler.vi"("error in (no error)"=w4) -> ()  [unwired: 4 in, 5 out]
